vi "API Send Debug Logger.vi"(9 "Response":string, 10 "Command":string, 11 "TimeToResponse":i32) -> (3 "Logged Responses":T1(array[cluster]))   [LabVIEW 2011]
panel:
  in  "Log responses longer than (ms)":i32=10000
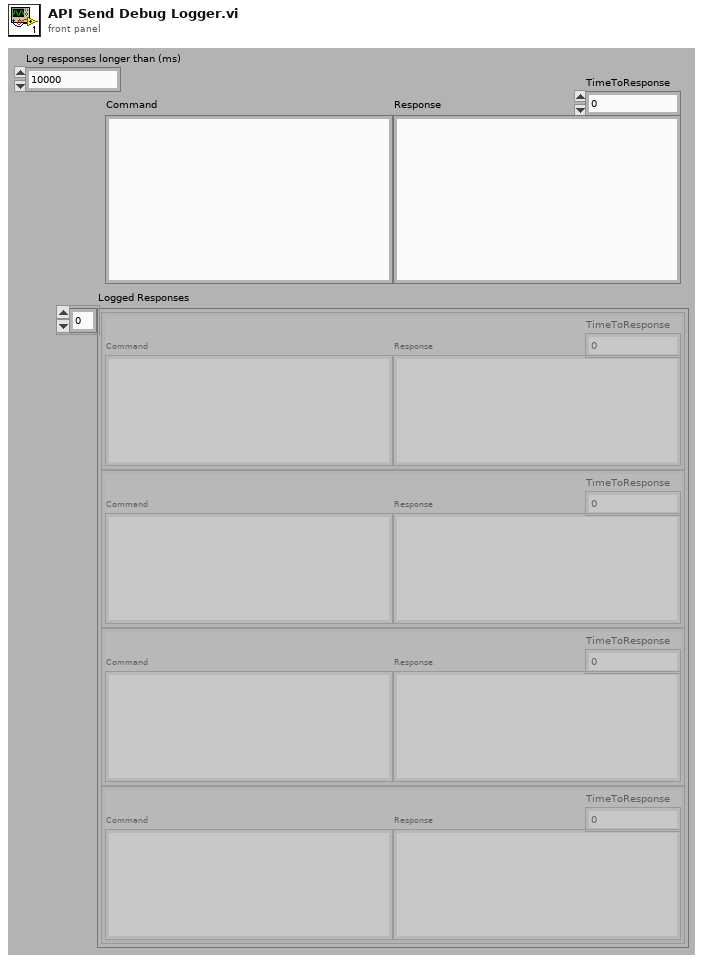
[diagram p1: front panel]
types:
  T1 = cluster{"TimeToResponse":i32, "Command":string, "Response":string}[]
  T2 = cluster{"TimeToResponse":i32, "Command":string, "Response":string}
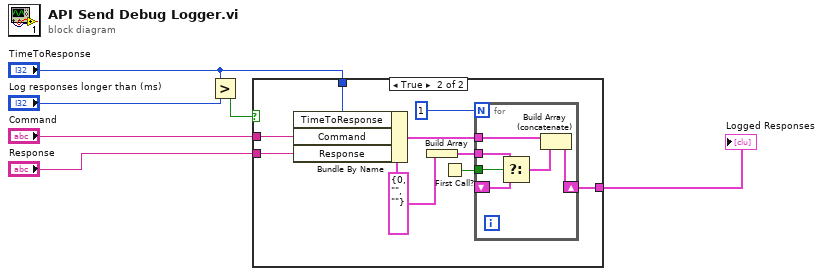
[diagram p0: block diagram]
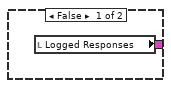
[diagram p2: hidden frame]
diagram:
  n1 = Greater?(x="TimeToResponse", y="Log responses longer than (ms)") -> (0:w2:bool)
  n2 = case shown="True" w2 {
    tunnel: "TimeToResponse" -> [_ w16]
    tunnel: "Command" -> [_ w15]
    tunnel: "Response" -> [_ w14]
    tunnel: [w7 w9] -> w1
    frame False {
      n3 = local read "Logged Responses"() -> (w7:T1)
    }
    frame True {
      w11 = T2 {"TimeToResponse"=0, "Command"="", "Response"=""} ("Logged Response")
      n4 = Bundle By Name(cluster=w11, "TimeToResponse"=w16, "Command"=w15, "Response"=w14) -> (w13:T2)
      n5 = Build Array(w11) -> (w10:T1)
      n6 = First Call?() -> (First Call?: T/F=w8:bool)
      n7 = for {
        N: 1 -> [_]
        tunnel: w13 -> [w22]
        shift-right: [w21] -> w9
        shift-left: _ -> [w17]
        tunnel: w8 -> [w20]
        tunnel: w10 -> [w19]
        n8 = Select(t=w19, s=w20, f=w17) -> (s? t:f=w18:T1)
        n9 = Build Array (concatenate)(w22, w18) -> (w21:T1)
      }
    }
  }
  "Logged Responses" <- w1
